vi "upperAngle calculator para Mantis.vi"(11 "Height to reach":dbl) -> (0 "Lower Angle":dbl, 3 "Upper Angle":dbl)   [LabVIEW 2015]
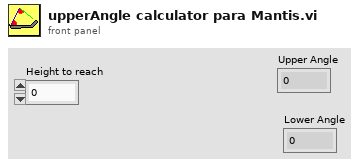
[diagram p1: front panel]
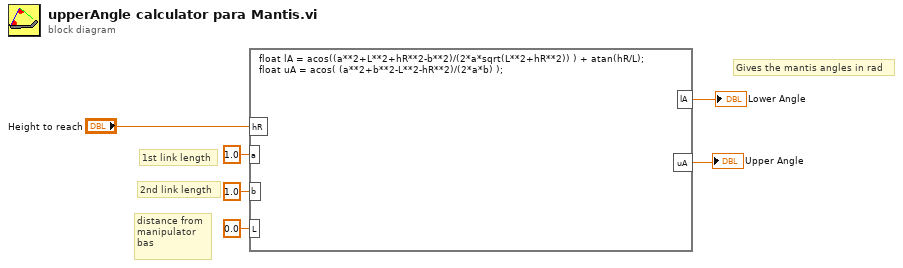
[diagram p0: block diagram]
diagram:
  # "Gives the mantis angles in rad"
  # "distance from\nmanipulator\nbas"
  # "2nd link length"
  # "1st link length"
  n1 = formula code="float lA = acos((a**2+L**2+hR**2-b**2)/(2*a*sqrt(L**2+hR**2)) ) + atan(hR/L);\nfloat uA = acos( (a**2+b**2-L**2-hR**2)/(2*a*b) );"("hR"="Height to reach", "a"=1.0 ("input variable"), "b"=1.0 ("input variable"), "L"=0.0 ("input variable")) -> ("lA"=→"Lower Angle":dbl, "uA"=→"Upper Angle":dbl)
